vi "Dt_to_kmH.vi"(11 "dt in":u32) -> (3 "Velocity (Km/h)":dbl)   [LabVIEW 2016]
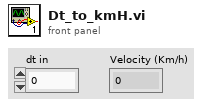
[diagram p1: front panel]
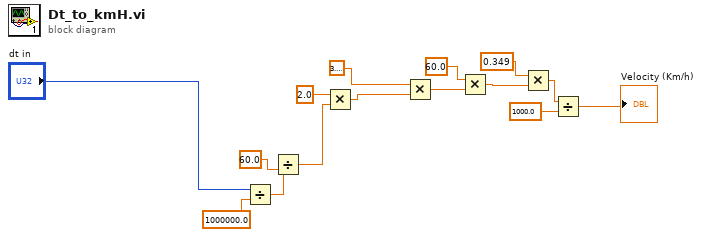
[diagram p0: block diagram]
diagram:
  n1 = Divide(x="dt in", y=1000000.0) -> (x/y=w7:dbl)
  n2 = Divide(x=w7, y=60.0 ("x")) -> (x/y=w2:dbl)
  n3 = Multiply(x=2.0, y=w2) -> (x*y=w4:dbl)
  n4 = Multiply(x=3.141592653589793, y=w4) -> (x*y=w9:dbl)
  n5 = Multiply(x=60.0, y=w9) -> (x*y=w11:dbl)
  n6 = Multiply(x=0.349, y=w11) -> (x*y=w13:dbl)
  n7 = Divide(x=w13, y=1000.0) -> (x/y=→"Velocity (Km/h)":dbl)
